vi "Open.vi"   [LabVIEW 2021, in "Field_RnD_Services_LIBSSH2_Toolkit.lvlib" / "SFTP Directory.lvclass"]
doc: "Creates a new SFTP Directory object that represents a libssh2lv shared library SFTP Directory struct. This VI must be called, or executed, before using any other SFTP Attributes-related VIs. This VI allocates memory within the libssh2lv shared library that must be explicitly deallocated, or freed, at the end of the application using the <B>Close</B> VI to avoid memory leaks or running Out-of-Memory (OOM) on a resource contrained system.\n\nA SFTP Directory object represents an existing directory, a.k.a. folder, on a remote SFTP filesystem."
uses:
  SFTP Directory.lvclass
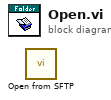
[diagram p0: block diagram]
diagram:
  n1 = call "Open from SFTP.vi"() -> ()  [unwired: 10 in, 2 out]
